vi "Visualization.vi"() -> ()   [LabVIEW 2014]
uses:
  <vilib>/Platform/TimedLoop/XDataNode/timing_clust.ctl
  <vilib>/Platform/TimedLoop/XDataNode/nitl_modes.ctl
  <vilib>/Platform/TimedLoop/XDataNode/wakeup.ctl
  <vilib>/Rock Robotics/Network Tables/SD Read Number.vi
  <vilib>/picture/3D Picture Control/Object/Create Object (drawable).vi
  <vilib>/platform/TimedLoop/XDataNode/XDataNode.xnode
  <vilib>/picture/3D Picture Control/NI_3D Picture Control.lvlib
  <vilib>/Platform/TimedLoop/XDataNode/XDNodeRunTimeDep.lvlib
panel:
  out "Gyro Display":refnum<vi>(3d-picture)
  in  "ref x 2":dbl format="%#_13g"
  in  "ref z 2":dbl format="%#_13g"
  in  "ref y 2":dbl format="%#_13g"
  out "Roll":dbl=0.4375
  out "Yaw":dbl=1.3125
  out "Pitch":dbl=0.125
  out "Z":dbl=0.125
  out "Y":dbl=1.3125
  out "X":dbl=0.4375
  in  "Set":bool
  in  "ref z":dbl format="%#_13g"
  in  "ref y":dbl format="%#_13g"
  in  "ref x":dbl format="%#_13g"
  in  "Period":i64=30
  out "Late?":bool=TRUE
  out "Fusion Display":refnum<vi>(3d-picture)
  in  "Length X":sgl=50.0
  in  "Length Z":sgl=30.0
  in  "Length Y":sgl=10.0
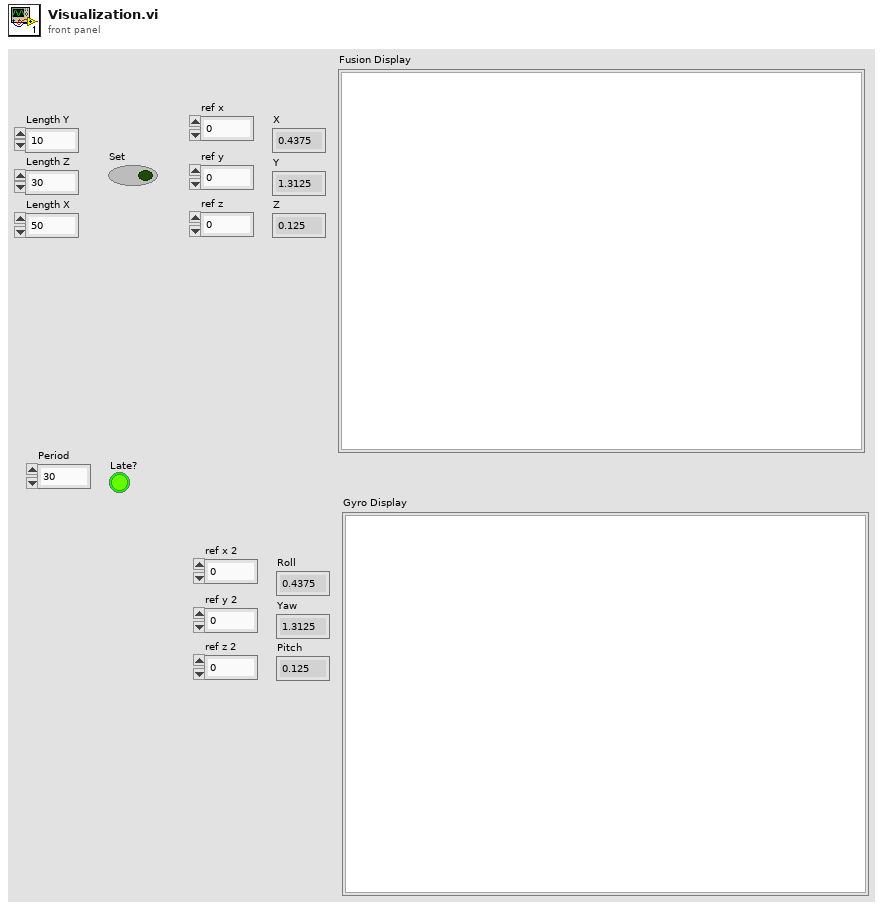
[diagram p1: front panel]
types:
  T1 = typedef "XDNodeRunTimeDep.lvlib/timing_clust.ctl" = cluster{"Expected End [f-1]":u64, "Actual End [f-1]":u64, "Finished Late? [f-1]":bool, "Expected End [i-1]":u64, "Actual End [i-1]":u64, "Finished Late? [i-1]":bool, "Expected Start [i]":u64, "Actual Start [i]":u64, "Expected Start [f]":u64, "Actual Start [f]":u64, "Source Name":string, "Structure Name":string, "Period":i64, "Deadline":i64, "Offset":i64, "Start":i64, "Priority":i32, "Timeout":i32, "Mode":T2, "Wakeup Reason":T3, "Error":errorcluster, "Source Type":string, "Secondary Source Type":string, "Global End Time":u64, "Global Start Time":u64, "Frame Duration":u64, "Iteration Duration":u64, "Assigned CPU":i32, "I/O Scan Engine Mode":u32}
  T2 = typedef "XDNodeRunTimeDep.lvlib/nitl_modes.ctl" = enum32{"No Change", "Process missed periods, maintain original phase", "Discard missed periods, maintain original phase", "Process missed periods, ignore original phase", "Discard missed periods, ignore original phase"}
  T3 = typedef "XDNodeRunTimeDep.lvlib/wakeup.ctl" = enum32{"Normal", "Aborted", "Asynchronous wakeup", "Timing source error", "Timed loop error", "Timeout"}
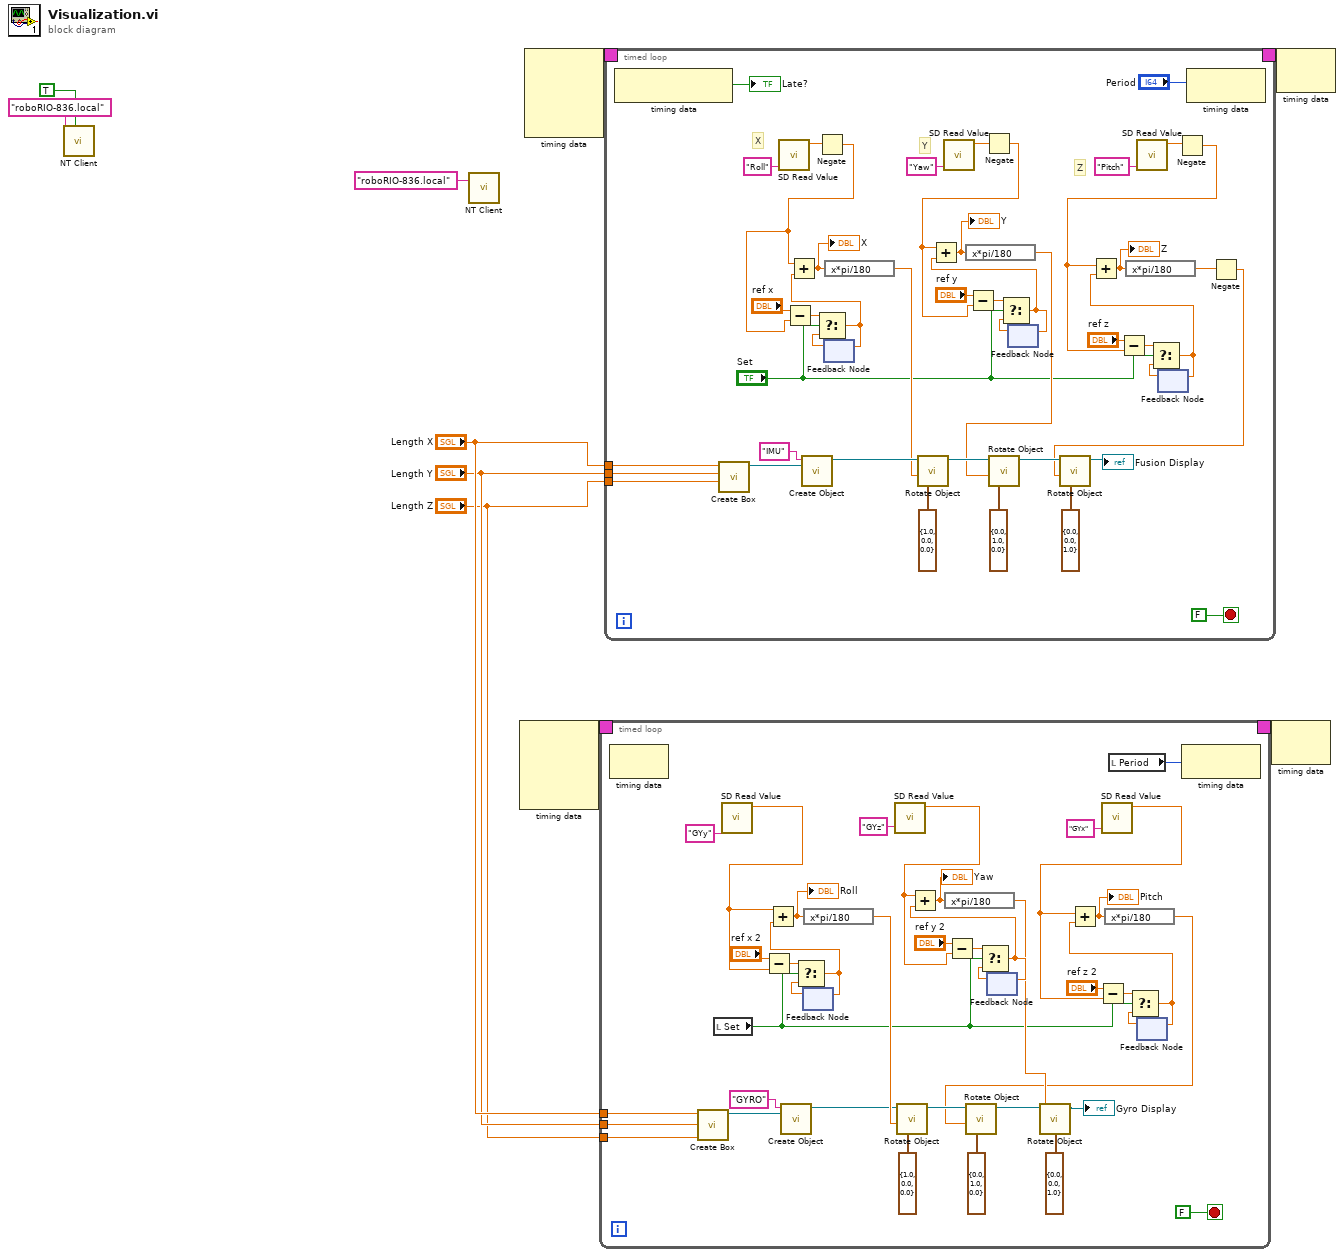
[diagram p0: block diagram]
diagram:
  n1 = call <vilib>:"NT Client.vi"("Automatic restart"=TRUE, "Server IP Address"="roboRIO-836.local") -> ()  [unwired: 10 in]
  n2 = call <vilib>:"NT Client.vi"("Server IP Address"="roboRIO-836.local") -> ()  [unwired: 11 in]
  n3 = node-c288() -> (w6:T1)  [unwired: 4 in]
  n4 = node-c288() -> (w8:T1)  [unwired: 4 in]
  n5 = timed-loop {
    timing: w6 -> [_]
    timing-out: [_] -> w5
    tunnel: "Length Y" -> [w21]
    tunnel: "Length X" -> [w20]
    tunnel: "Length Z" -> [w19]
    stop <- FALSE stop-if-true
    n6 = node-c288() -> ()  [unwired: 1 in, 1 out]
    n7 = call <vilib>:"Create Box.vi"("Length Z"=w19, "Length Y"=w21, "Length X"=w20) -> ("New Box Refnum"=w32:refnum<vi>)  [unwired: 7 in, 1 out]
    n8 = local read "Set"() -> (w12:bool)
    n9 = call-poly <vilib>:"SD Read Value.vi"("Name"="GYy") -> ("Numeric"=w17:dbl)  [unwired: 8 in, 2 out]
    n10 = Subtract(x="ref x 2", y=w17) -> (x-y=w35:dbl)
    n11 = call-poly <vilib>:"Create Object.vi"("Geometry"=w32, "Name"="GYRO") -> ("Scene:New Object"=w31:refnum<vi>)  [unwired: 8 in, 1 out]
    n12 = feedback #1() -> (w37:dbl)  [unwired: 1 in]
    n13 = Select(t=w35, s=w12, f=w37) -> (s? t:f=w36:dbl)
    n14 = Add(x=w17, y=w36) -> (x+y=w46:dbl)
    "Roll" <- w46
    n15 = feedback-in #1(w36) -> ()
    n16 = expression code="x*pi/180"(w46) -> (w33:dbl)
    n17 = call-poly <vilib>:"SD Read Value.vi"("Name"="GYz") -> ("Numeric"=w16:dbl)  [unwired: 8 in, 2 out]
    n18 = call <vilib>:"Rotate Object.vi"("Angle"=w33, "Axis"=cluster{"X":sgl, "Y":sgl, "Z":sgl} {"X"=1.0, "Y"=0.0, "Z"=0.0}, "Scene.Object In"=w31) -> ("Scene.Object Out"=w28:refnum<vi>)  [unwired: 7 in, 1 out]
    n19 = Subtract(x="ref y 2", y=w16) -> (x-y=w40:dbl)
    n20 = feedback #2() -> (w41:dbl)  [unwired: 1 in]
    n21 = Select(t=w40, s=w12, f=w41) -> (s? t:f=w45:dbl)
    n22 = Add(x=w16, y=w45) -> (x+y=w47:dbl)
    "Yaw" <- w47
    n23 = expression code="x*pi/180"(w47) -> (w14:dbl)
    n24 = feedback-in #2(w45) -> ()
    n25 = call-poly <vilib>:"SD Read Value.vi"("Name"="GYx") -> ("Numeric"=w15:dbl)  [unwired: 8 in, 2 out]
    n26 = Subtract(x="ref z 2", y=w15) -> (x-y=w43:dbl)
    n27 = local read "Period"() -> (w11:i64)
    n28 = feedback #3() -> (w42:dbl)  [unwired: 1 in]
    n29 = Select(t=w43, s=w12, f=w42) -> (s? t:f=w44:dbl)
    n30 = Add(x=w15, y=w44) -> (x+y=w48:dbl)
    "Pitch" <- w48
    n31 = expression code="x*pi/180"(w48) -> (w13:dbl)
    n32 = call <vilib>:"Rotate Object.vi"("Angle"=w13, "Axis"=cluster{"X":sgl, "Y":sgl, "Z":sgl} {"X"=0.0, "Y"=1.0, "Z"=0.0}, "Scene.Object In"=w28) -> ("Scene.Object Out"=w29:refnum<vi>)  [unwired: 7 in, 1 out]
    n33 = call <vilib>:"Rotate Object.vi"("Angle"=w14, "Axis"=cluster{"X":sgl, "Y":sgl, "Z":sgl} {"X"=0.0, "Y"=0.0, "Z"=1.0}, "Scene.Object In"=w29) -> ("Scene.Object Out"=→"Gyro Display":refnum<vi>)  [unwired: 7 in, 1 out]
    n34 = feedback-in #3(w44) -> ()
    n35 = node-c288(w11) -> ()  [unwired: 1 out]
  }
  n36 = timed-loop {
    tunnel: "Length X" -> [w82]
    tunnel: "Length Y" -> [w81]
    tunnel: "Length Z" -> [w80]
    timing: w8 -> [_]
    timing-out: [_] -> w7
    stop <- FALSE stop-if-true
    # "Y"
    # "X"
    # "Z"
    n37 = node-c288() -> (→"Late?":bool)  [unwired: 1 in]
    n38 = call <vilib>:"Create Box.vi"("Length Z"=w80, "Length Y"=w81, "Length X"=w82) -> ("New Box Refnum"=w88:refnum<vi>)  [unwired: 7 in, 1 out]
    n39 = call-poly <vilib>:"SD Read Value.vi"("Name"="Roll") -> ("Numeric"=w58:dbl)  [unwired: 8 in, 2 out]
    n40 = call-poly <vilib>:"Create Object.vi"("Geometry"=w88, "Name"="IMU") -> ("Scene:New Object"=w89:refnum<vi>)  [unwired: 8 in, 1 out]
    n41 = Negate(x=w58) -> (-x=w56:dbl)
    n42 = Subtract(x="ref x", y=w56) -> (x-y=w76:dbl)
    n43 = feedback #4() -> (w74:dbl)  [unwired: 1 in]
    n44 = Select(t=w76, s="Set", f=w74) -> (s? t:f=w75:dbl)
    n45 = Add(x=w56, y=w75) -> (x+y=w64:dbl)
    "X" <- w64
    n46 = feedback-in #4(w75) -> ()
    n47 = expression code="x*pi/180"(w64) -> (w84:dbl)
    n48 = call <vilib>:"Rotate Object.vi"("Angle"=w84, "Axis"=cluster{"X":sgl, "Y":sgl, "Z":sgl} {"X"=1.0, "Y"=0.0, "Z"=0.0}, "Scene.Object In"=w89) -> ("Scene.Object Out"=w92:refnum<vi>)  [unwired: 7 in, 1 out]
    n49 = call-poly <vilib>:"SD Read Value.vi"("Name"="Yaw") -> ("Numeric"=w93:dbl)  [unwired: 8 in, 2 out]
    n50 = Negate(x=w93) -> (-x=w55:dbl)
    n51 = Subtract(x="ref y", y=w55) -> (x-y=w71:dbl)
    n52 = feedback #5() -> (w70:dbl)  [unwired: 1 in]
    n53 = Select(t=w71, s="Set", f=w70) -> (s? t:f=w66:dbl)
    n54 = Add(x=w55, y=w66) -> (x+y=w63:dbl)
    "Y" <- w63
    n55 = expression code="x*pi/180"(w63) -> (w83:dbl)
    n56 = call <vilib>:"Rotate Object.vi"("Angle"=w83, "Axis"=cluster{"X":sgl, "Y":sgl, "Z":sgl} {"X"=0.0, "Y"=1.0, "Z"=0.0}, "Scene.Object In"=w92) -> ("Scene.Object Out"=w91:refnum<vi>)  [unwired: 7 in, 1 out]
    n57 = feedback-in #5(w66) -> ()
    n58 = call-poly <vilib>:"SD Read Value.vi"("Name"="Pitch") -> ("Numeric"=w59:dbl)  [unwired: 8 in, 2 out]
    n59 = feedback #6() -> (w69:dbl)  [unwired: 1 in]
    n60 = Negate(x=w59) -> (-x=w57:dbl)
    n61 = Subtract(x="ref z", y=w57) -> (x-y=w68:dbl)
    n62 = Select(t=w68, s="Set", f=w69) -> (s? t:f=w67:dbl)
    n63 = Add(x=w57, y=w67) -> (x+y=w62:dbl)
    "Z" <- w62
    n64 = expression code="x*pi/180"(w62) -> (w61:dbl)
    n65 = feedback-in #6(w67) -> ()
    n66 = node-c288("Period") -> ()  [unwired: 1 out]
    n67 = Negate(x=w61) -> (-x=w60:dbl)
    n68 = call <vilib>:"Rotate Object.vi"("Angle"=w60, "Axis"=cluster{"X":sgl, "Y":sgl, "Z":sgl} {"X"=0.0, "Y"=0.0, "Z"=1.0}, "Scene.Object In"=w91) -> ("Scene.Object Out"=→"Fusion Display":refnum<vi>)  [unwired: 7 in, 1 out]
  }
  n69 = node-c288(w5) -> ()  [unwired: 1 out]
  n70 = node-c288(w7) -> ()  [unwired: 1 out]
